vi "GetVIPanesAndSplitters.vi"(0 "path":path, 11 "error in (no error)":errorcluster) -> (2 "Front Panel":refnum<vi>, 3 "Vertical Splitters On top?":bool, 4 "Splitters":T3, 6 "Panes":T4, 8 "Splitters Widths":T2, 10 "Colors":T1, 12 "Number of Splitters":i32, 14 "vi reference":refnum<vi>, 15 "error out":errorcluster)   [LabVIEW 2022 SP3, in "PentaPanesLibrary.lvlib" / "PentaPanes.lvclass"]
uses:
  PentaPanes.lvclass
  PanesCluster.ctl
  SplittersCluster.ctl
  SplittersWidthCluster.ctl
  PanesColors.ctl
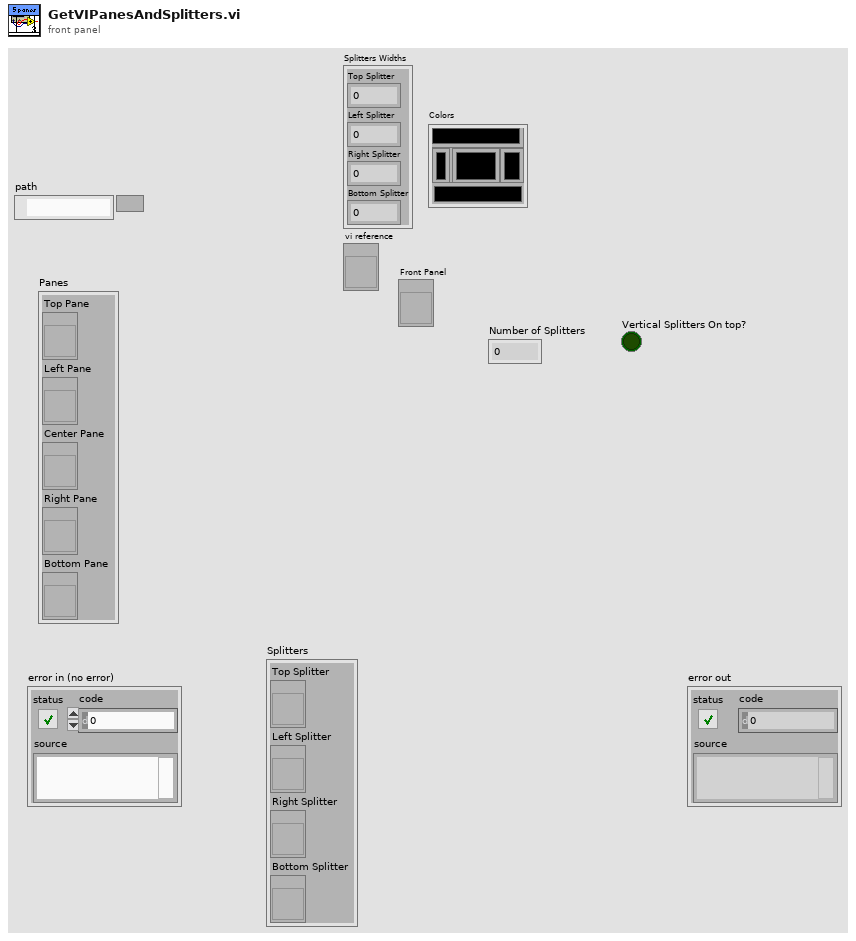
[diagram p1: front panel]
types:
  T1 = typedef "PentaPanesLibrary.lvlib/PentaPanes.lvclass/PanesColors.ctl" = cluster{"Top Color":u32, "Left Color":u32, "Center Color":u32, "Right Color":u32, "Bottom Color":u32}
  T2 = typedef "PentaPanesLibrary.lvlib/PentaPanes.lvclass/SplittersWidthCluster.ctl" = cluster{"Top Splitter":i32, "Left Splitter":i32, "Right Splitter":i32, "Bottom Splitter":i32}
  T3 = typedef "PentaPanesLibrary.lvlib/PentaPanes.lvclass/SplittersCluster.ctl" = cluster{"Top Splitter":refnum<vi>, "Left Splitter":refnum<vi>, "Right Splitter":refnum<vi>, "Bottom Splitter":refnum<vi>}
  T4 = typedef "PentaPanesLibrary.lvlib/PentaPanes.lvclass/PanesCluster.ctl" = cluster{"Top Pane":refnum<vi>, "Left Pane":refnum<vi>, "Center Pane":refnum<vi>, "Right Pane":refnum<vi>, "Bottom Pane":refnum<vi>}
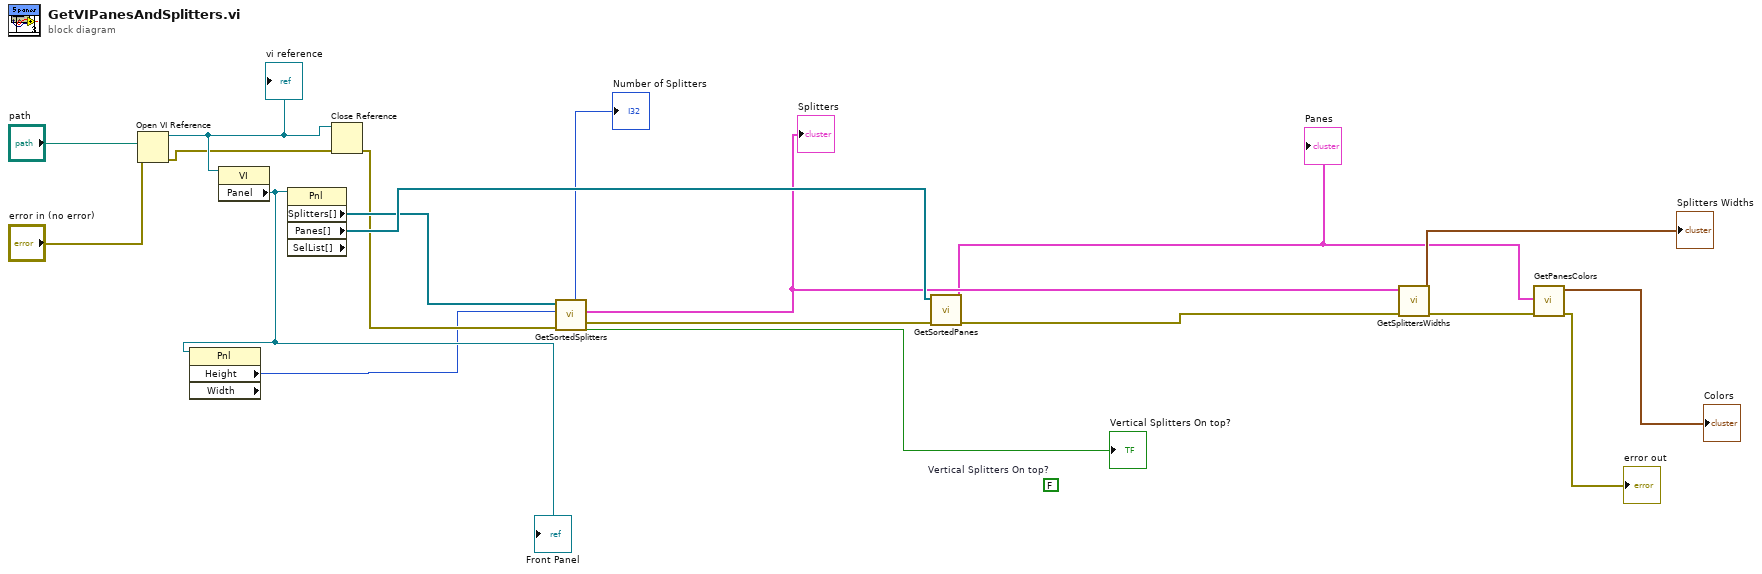
[diagram p0: block diagram]
diagram:
  (unwired) FALSE  # Vertical Splitters On top?
  n1 = Open VI Reference(vi path="path", error in (no error)="error in (no error)") -> (vi reference=w16:refnum<vi>, error out=w15:errorcluster)  [unwired: 4 in]
  "vi reference" <- w16
  n2 = property class="VI"(reference=w16) -> ("Panel"=w12:refnum<vi>)  [unwired: 1 in, 2 out]
  "Front Panel" <- w12
  n3 = property class="Pnl" props=["Height", "Width"](reference=w12) -> ("Height"=w11:u32)  [unwired: 1 in, 3 out]
  n4 = property class="Pnl" props=["Splitters[]", "Panes[]", "SelList[]"](reference=w12) -> ("Splitters[]"=w18:refnum<vi>[], "Panes[]"=w19:refnum<vi>[])  [unwired: 1 in, 3 out]
  n5 = Close Reference(reference=w16, error in (no error)=w15) -> (error out=w14:errorcluster)
  n6 = call "GetSortedSplitters.vi"("error in (no error)"=w14, "Height"=w11, "Splitters[]"=w18) -> ("error out"=w13:errorcluster, "Splitters"=w7:T3, "Vertical on Top?"=→"Vertical Splitters On top?":bool, "Number of Splitters"=→"Number of Splitters":i32)  [unwired: 3 in, 2 out]
  "Splitters" <- w7
  n7 = call "GetSortedPanes.vi"("error in (no error)"=w13, "Panes[]"=w19) -> ("error out"=w4:errorcluster, "Panes"=w2:T4)  [unwired: 8 in]
  "Panes" <- w2
  n8 = call "GetSplittersWidths.vi"("error in (no error)"=w4, "Splitters"=w7) -> ("error out"=w5:errorcluster, "Splitters Widths"=→"Splitters Widths":T2)  [unwired: 8 in]
  n9 = call "GetPanesColors.vi"("error in (no error)"=w5, "Panes"=w2) -> ("error out"=→"error out":errorcluster, "Colors"=→"Colors":T1)  [unwired: 8 in]
